vi "Write AI.vi"(0 "OPC UA server refnum in":T3, 1 "AI":T1, 2 "AI tags":string[](array[string]), 5 "error in (no error)":errorcluster, 6 "OPC UA AI list":string[](array[string])) -> (14 "OPC UA server refnum out":T3, 19 "error out":errorcluster)   [LabVIEW 2019, in "OPC addons.lvlib"]
uses:
  OPC addons.lvlib
  <vilib>/OPCUA/controls/OPC UA Server Refnum.ctl
  Inputs/Ctl/AI short.ctl
  Inputs/Ctl/Parameter State.ctl
  <vilib>/OPCUA/controls/Write Status.ctl
  <vilib>/OPCUA/server/Write Variant.vi
  <vilib>/OPCUA/NI OPC UA Server.lvlib
  Inputs/Inputs.lvlib
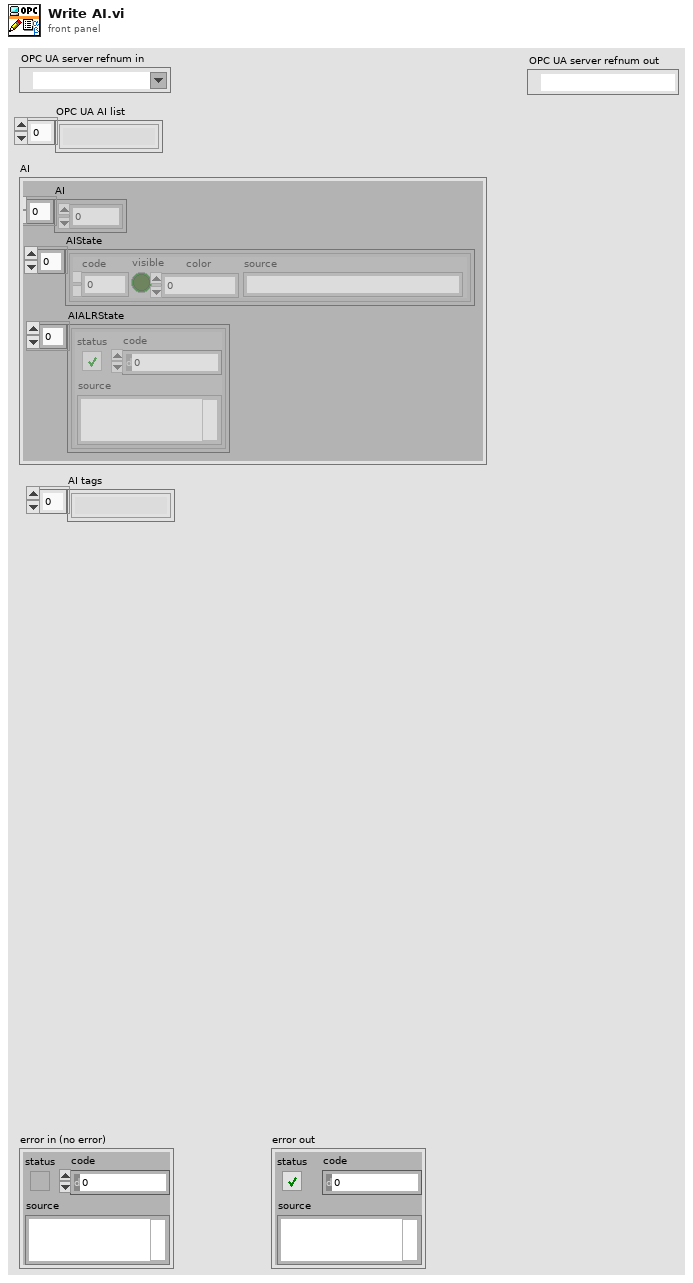
[diagram p1: front panel]
types:
  T1 = typedef "Inputs.lvlib/AI short.ctl" = cluster{"AI":dbl[], "AIState":T2[], "AIALRState":errorcluster[]}
  T2 = typedef "Inputs.lvlib/Parameter State.ctl" = cluster{"code":i32, "visible":bool, "color":u32, "source":string}
  T3 = typedef "OPC UA Server Refnum.ctl" = refnum<k21>
  T4 = typedef "Write Status.ctl" = u32
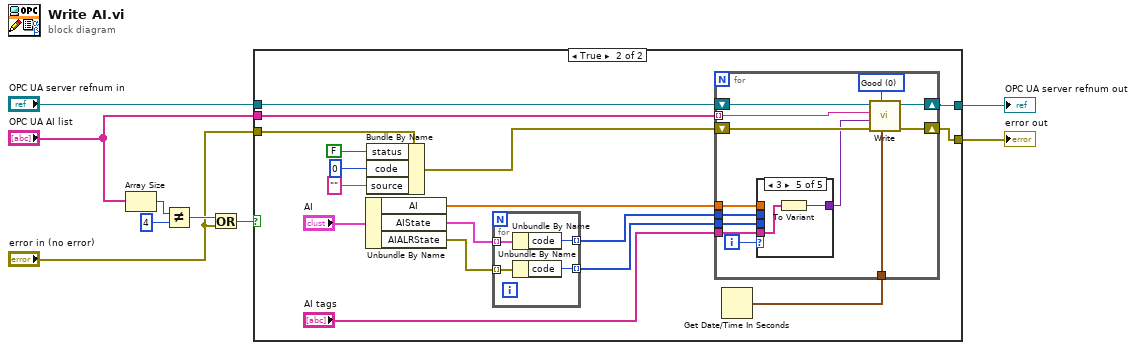
[diagram p0: block diagram]
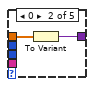
[diagram p4: hidden frame]
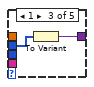
[diagram p5: hidden frame]
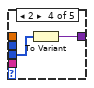
[diagram p6: hidden frame]
diagram:
  n1 = Array Size(array="OPC UA AI list") -> (size(s)=w5:i32)
  n2 = Not Equal?(x=w5, y=4) -> (x != y?=w3:bool)
  n3 = Or(x=w3, y="error in (no error)") -> (x .or. y?=w1:bool)
  n4 = case shown="True" w1 {
    tunnel: "OPC UA server refnum in" -> [w11 w21]
    tunnel: [w11 w20] -> w8
    tunnel: [w10 w19] -> w7
    tunnel: "OPC UA AI list" -> [_ w17]
    tunnel: "error in (no error)" -> [w10 w16]
    frame False {
    }
    frame True {
      n5 = Unbundle By Name("AI") -> ("AI"=w26:dbl[], "AIState"=w27:T2[], "AIALRState"=w28:errorcluster[])
      n6 = Bundle By Name(cluster=w16, "status"=FALSE, "code"=0, "source"="") -> (w15:errorcluster)
      n7 = for {
        tunnel: w27 -> [w53] mode=indexing
        tunnel: [w52] -> w23 mode=indexing
        tunnel: w28 -> [w51] mode=indexing
        tunnel: [w50] -> w24 mode=indexing
        n8 = Unbundle By Name(w53) -> ("code"=w52:i32)
        n9 = Unbundle By Name(w51) -> ("code"=w50:i32)
      }
      n10 = Get Date/Time In Seconds() -> (seconds since 1Jan1904=w22:timestamp)
      n11 = for {
        tunnel: w22 -> [w33]
        tunnel: w26 -> [w41]
        tunnel: w23 -> [w39]
        tunnel: w17 -> [w31] mode=indexing
        tunnel: w24 -> [w38]
        tunnel: "AI tags" -> [w37]
        shift-right: [w30] -> w20
        shift-left: w21 -> [w35]
        shift-right: [w29] -> w19
        shift-left: w15 -> [w34]
        i -> [w40]
        w36 = T4 0 items=["Good"=0, "Uncertain"=1073741824, "Uncertain_InitialValue"=1083310080, "Uncertain_LastUsableValue"=1083179008, "Uncertain_SensorNotAccurate"=1083375616, "Uncertain_EngineeringUnitsExceeded"=1083441152, "Bad"=2147483648, "Bad_NoCommunication"=2150694912, "Bad_NotReadable"=2151284736, "Bad_NotWritable"=2151350272, "Bad_OutOfRange"=2151415808, "Bad_WaitingForInitialData"=2150760448] ("node status")
        n12 = case shown="3" w40 {
          tunnel: w41 -> [_ w43 _ _ _]
          tunnel: [_ w42 w45 w47 w49] -> w32
          tunnel: w39 -> [_ _ w44 _ _]
          tunnel: w38 -> [_ _ _ w46 _]
          tunnel: w37 -> [_ _ _ _ w48]
          frame -1, Default {
          }
          frame 0 {
            n13 = To Variant(anything=w43) -> (Variant=w42:variant)
          }
          frame 1 {
            n14 = To Variant(anything=w44) -> (Variant=w45:variant)
          }
          frame 2 {
            n15 = To Variant(anything=w46) -> (Variant=w47:variant)
          }
          frame 3 {
            n16 = To Variant(anything=w48) -> (Variant=w49:variant)
          }
        }
        n17 = call-poly <vilib>:"Write.vi"("timestamp (current time)"=w33, "node status"=w36, "error in (no error)"=w34, "value"=w32, "node ID"=w31, "OPC UA server refnum in"=w35) -> ("error out"=w29:errorcluster, "OPC UA server refnum out"=w30:T3)  [unwired: 3 in, 1 out]
      }
    }
  }
  "OPC UA server refnum out" <- w8
  "error out" <- w7
